vi "MDAQ_SpectrumLoad.vi"(8 "error in":errorcluster, 9 "Status_Cluster":T1 {"GATESTOP" format="%04x"; "GATESTRT" format="%04x"; "AMPLITUDE" format="%04x"; "M_CYCLES" format="%04x"; "N_CYCLES" format="%04x"; "STEP" format="%04x"; "BASE" format="%04x"; "CHAN" format="%04x"}) -> (0 "error IO":errorcluster, 1 "Status_Cluster Out":T1 {"GATESTOP" format="%04x"; "GATESTRT" format="%04x"; "AMPLITUDE" format="%04x"; "M_CYCLES" format="%04x"; "N_CYCLES" format="%04x"; "STEP" format="%04x"; "BASE" format="%04x"; "CHAN" format="%04x"})   [LabVIEW 2021]
uses:
  Status_Cluster.ctl
  <vilib>/regexp/Match Regular Expression.xnode
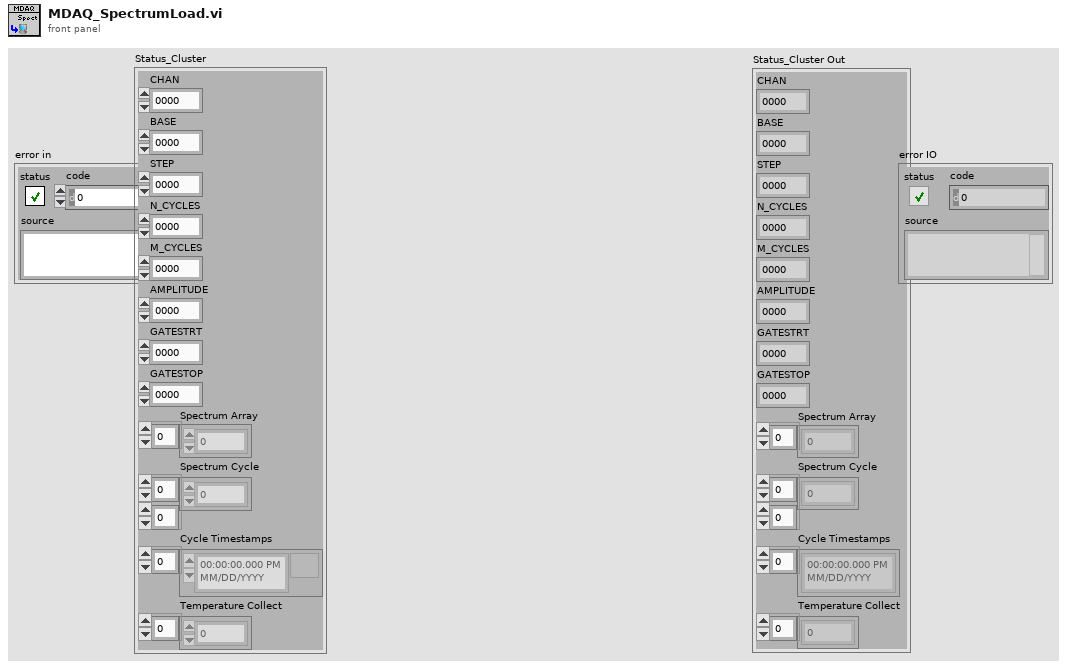
[diagram p1: front panel]
types:
  T1 = typedef "Status_Cluster.ctl" = cluster{"CHAN":u32, "BASE":u32, "STEP":u32, "N_CYCLES":u32, "M_CYCLES":u32, "AMPLITUDE":u32, "GATESTRT":u32, "GATESTOP":u32, "Spectrum Array":u32[], "Spectrum Cycle":u32[][], "Cycle Timestamps":timestamp[], "Temperature Collect":dbl[]}
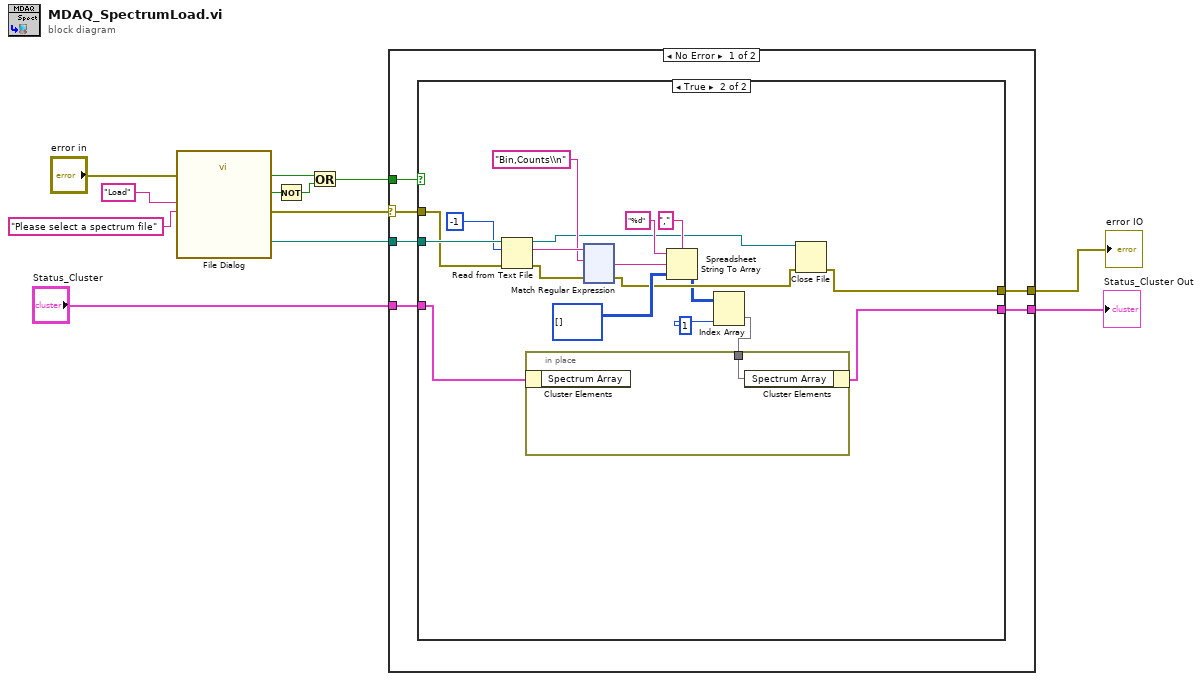
[diagram p0: block diagram]
diagram:
  n1 = call "File Dialog"("prompt"="Please select a spectrum file", "button label"="Load", "error in"="error in") -> ("selected path"=w6:path, "exists"=w9:bool, "cancelled"=w4:bool, "error out"=w8:errorcluster)  [unwired: 9 in]
  n2 = Not(x=w4) -> (.not. x?=w5:bool)
  n3 = Or(x=w9, y=w5) -> (x .or. y?=w7:bool)
  n4 = case shown="No Error" w8 {
    selector: w8 -> [w15 w158]
    tunnel: w7 -> [w18 _]
    tunnel: w6 -> [w17 _]
    tunnel: "Status_Cluster" -> [w16 w157]
    tunnel: [w14 w158] -> w1
    tunnel: [w13 w157] -> w2
    frame No Error {
      n5 = case shown="True" w18 {
        tunnel: w17 -> [_ w38]
        tunnel: w16 -> [w19 w28]
        tunnel: w15 -> [w20 w36]
        tunnel: [w20 w24] -> w14
        tunnel: [w19 w27] -> w13
        frame False {
        }
        frame True {
          n6 = Read from Text File(file (use dialog)=w38, count=-1, error in=w36) -> (refnum out=w26:refnum<file>, text=w35:string, error out=w34:errorcluster)  [unwired: 1 in, 1 out]
          n7 = xnode "Match Regular Expression"("input string"=w35, "regular expression"="Bin,Counts\\n", "error in"=w34) -> ("after match"=w32:string, "error out"=w25:errorcluster)  [unwired: 3 in, 3 out]
          n8 = Spreadsheet String To Array(delimiter (Tab)=",", format string="%d", spreadsheet string=w32, array type (2D Dbl)=u32[][] []) -> (array=w23:u32[][])
          n9 = Index Array(array=w23, index (col)=1 ("disabled index (col)")) -> (element=w21:u32[])  [unwired: 1 in]
          n10 = in-place {
            in-place-border: w21 -> [w39]
            n11 = in-place-cluster #1(w28) -> ()  [unwired: 1 out]
            n12 = in-place-cluster #1("Spectrum Array"=w39) -> (w27:T1)
          }
          n13 = Close File(refnum=w26, error in=w25) -> (error out=w24:errorcluster)  [unwired: 1 out]
        }
      }
    }
    frame Error {
    }
  }
  "Status_Cluster Out" <- w2
  "error IO" <- w1
